vi "Channel Stop.vi"(8 "error in (no error)":errorcluster, 10 "Channel Index":i32, 11 "Mixer in":refnum<class "Mixer.lvclass">) -> (0 "error out":errorcluster, 3 "Mixer out":refnum<class "Mixer.lvclass">)   [LabVIEW 2020, in "G-Audio.lvlib" / "Mixer.lvclass"]
uses:
  Mixer.lvclass
  Message.ctl
  Command.ctl
  Mixer.lvclass/Mixer.ctl
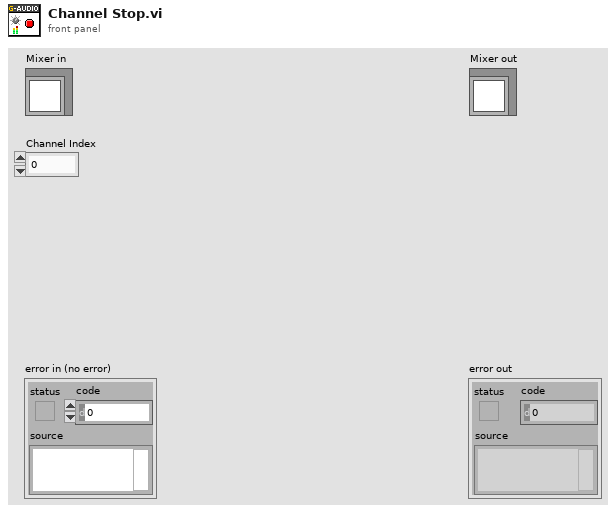
[diagram p1: front panel]
types:
  T1 = typedef "G-Audio.lvlib/Mixer.lvclass/Message.ctl" = cluster{"Command":T2, "Channel":i32, "Payload":variant}
  T2 = typedef "G-Audio.lvlib/Mixer.lvclass/Command.ctl" = enum16{"Channel Stop", "Channel Pause", "Channel Play", "Channel Volume"}
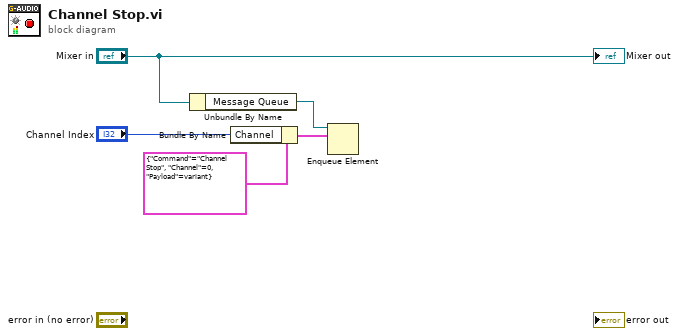
[diagram p0: block diagram]
diagram:
  n1 = Unbundle By Name("Mixer in") -> ("Message Queue"=w5:refnum<queue>)
  n2 = Bundle By Name(cluster=T1 {"Command"=enum."Channel Stop", "Channel"=0, "Payload"=variant} ("element"), "Channel"="Channel Index") -> (w3:T1)
  n3 = Enqueue Element(queue=w5, element=w3) -> ()  [unwired: 2 in, 3 out]
  "Mixer out" <- "Mixer in"
